vi "Starbuzz Coffee.vi"() -> ()   [LabVIEW 2017]
uses:
  Decaf/Decaf.lvclass
  C:/Users/fflores/Documents/LabVIEW-Open-Projects/LabIVEW OOP Design Patterns/Decorator Pattern/Starbuzz Coffee Example/Beverage Class/Beverage.lvclass
  Espresso/Espresso.lvclass
  HouseBlend/HouseBlend.lvclass
  DarkRoast/DarkRoast.lvclass
  MintTea/MintTea.lvclass
  Mocha/Mocha.lvclass
  C:/Users/fflores/Documents/LabVIEW-Open-Projects/LabIVEW OOP Design Patterns/Decorator Pattern/Starbuzz Coffee Example/CondimentDecorator/CondimentDecorator.lvclass
  Soy/Soy.lvclass
  Milk/Milk.lvclass
  CondimentDecorator/CondimentDecorator.lvclass
  Vanilla/Vanilla.lvclass
  Beverage Class/Beverage.lvclass
panel:
  in  "Beverage":T1(ring)
  in  "Topping":T2(ring)
  out "cost":dbl format="$ %#.3g"
  out "description":string
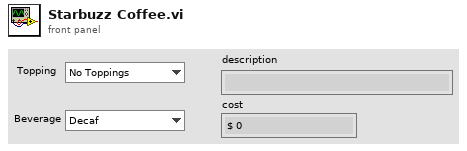
[diagram p1: front panel]
types:
  T1 = enum16{"Decaf", "Dark Roast", "MintTea", "Espresso", "House Blend"}
  T2 = enum16{"No Toppings", "Milk", "Vanilla", "Mocha", "Soy"}
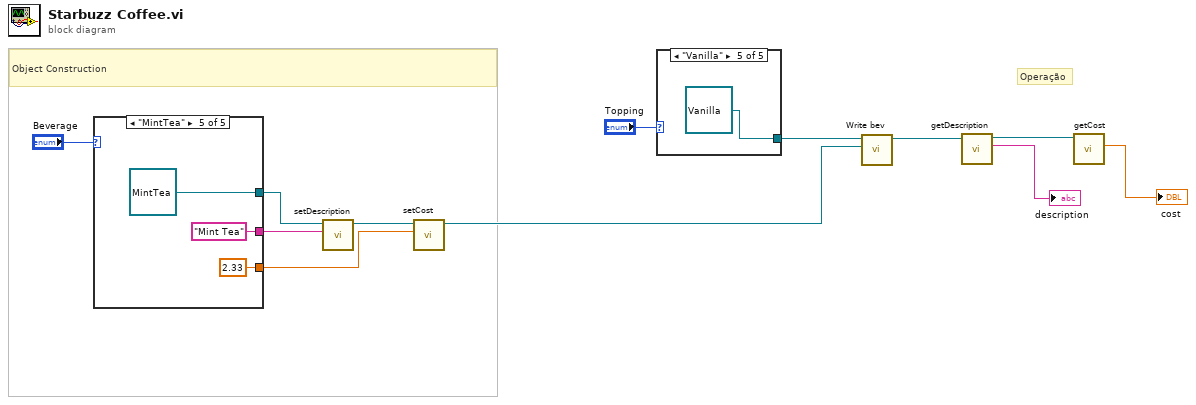
[diagram p0: block diagram]
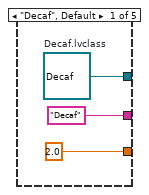
[diagram p2: hidden frame]
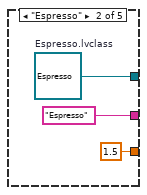
[diagram p3: hidden frame]
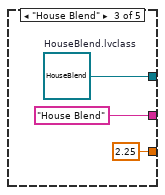
[diagram p4: hidden frame]
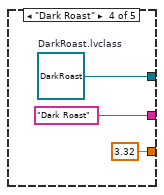
[diagram p5: hidden frame]
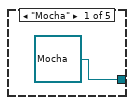
[diagram p6: hidden frame]
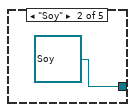
[diagram p7: hidden frame]
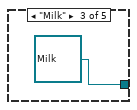
[diagram p8: hidden frame]
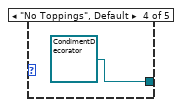
[diagram p9: hidden frame]
diagram:
  # "Operação"
  # "Object Construction"
  n1 = case shown="\"MintTea\"" "Beverage" {
    tunnel: [w15 w18 w21 w24 refnum<class "MintTea.lvclass"> refnum ("MintTea.lvclass")] -> w8
    tunnel: ["Decaf" "Espresso" "House Blend" "Dark Roast" "Mint Tea"] -> w7
    tunnel: [2.0 1.5 2.25 3.32 2.33] -> w2
    frame "Decaf", Default {
      w15 = refnum<class "Decaf.lvclass"> refnum  # Decaf.lvclass
    }
    frame "Espresso" {
      w18 = refnum<class "Espresso.lvclass"> refnum  # Espresso.lvclass
    }
    frame "House Blend" {
      w21 = refnum<class "HouseBlend.lvclass"> refnum  # HouseBlend.lvclass
    }
    frame "Dark Roast" {
      w24 = refnum<class "DarkRoast.lvclass"> refnum  # DarkRoast.lvclass
    }
    frame "MintTea" {
    }
  }
  n2 = call-dynamic "setDescription.vi"("description"=w7, "Beverage in"=w8) -> ("Beverage out"=w6:refnum<class "Beverage.lvclass">)  [unwired: 8 in, 1 out]
  n3 = call-dynamic "setCost.vi"("cost"=w2, "Beverage in"=w6) -> ("Beverage out"=w3:refnum<class "Beverage.lvclass">)  [unwired: 8 in, 1 out]
  n4 = case shown="\"Vanilla\"" "Topping" {
    tunnel: [refnum<class "Mocha.lvclass"> refnum ("Mocha.lvclass") refnum<class "Soy.lvclass"> refnum ("Soy.lvclass") refnum<class "Milk.lvclass"> refnum ("Milk.lvclass") refnum<class "CondimentDecorator.lvclass"> refnum ("CondimentDecorator.lvclass") refnum<class "Vanilla.lvclass"> refnum ("Vanilla.lvclass")] -> w4
    frame "Mocha" {
    }
    frame "Soy" {
    }
    frame "Milk" {
    }
    frame "No Toppings", Default {
    }
    frame "Vanilla" {
    }
  }
  n5 = call-dynamic "Write bev.vi"("Beverage.lvclass"=w3, "CondimentDecorator in"=w4) -> ("CondimentDecorator out"=w5:refnum<class "CondimentDecorator.lvclass">)  [unwired: 8 in, 1 out]
  n6 = call-dynamic "getDescription.vi"("CondimentDecorator in"=w5) -> ("description"=→"description":string, "CondimentDecorator out"=w1:refnum<class "CondimentDecorator.lvclass">)  [unwired: 8 in, 1 out]
  n7 = call-dynamic "getCost.vi"("CondimentDecorator in"=w1) -> ("cost"=→"cost":dbl)  [unwired: 8 in, 2 out]
